vi "gu_free.vi"(8 "error in":errorcluster, 11 "pointer":i64) -> (0 "error out":errorcluster)   [LabVIEW 2020, in "G-Unicode.lvlib"]
doc: "Free the memory pointed to by <b>pointer</b>."
uses:
  G-Unicode.lvlib
  lib/g_unicode_32.dll
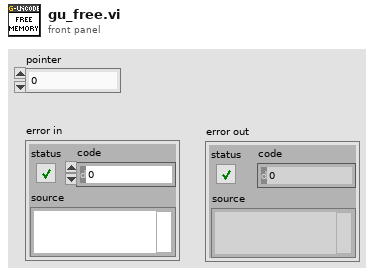
[diagram p1: front panel]
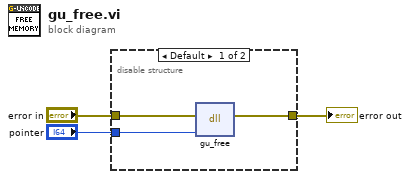
[diagram p0: block diagram]
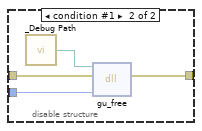
[diagram p2: hidden frame]
diagram:
  n1 = disable-structure shown="Default" {
    disable-tunnel: "pointer" -> [w6 w10]
    disable-tunnel: "error in" -> [w5 w9]
    disable-tunnel: [w4 w8] -> w1
    frame condition #0 (active) {
      n2 = dll-call lib="C:/github/dataflowg/g-unicode/src/LabVIEW/G-Unicode/lib/g_unicode_*.*" fn="gu_free"(error in=w5, "pointer"=w6) -> (error out=w4:errorcluster)  [unwired: 4 in, 1 out]
    }
    frame condition #1 {
      n3 = call "_Debug Path.vi"() -> ("Debug Path"=w7:path)
      n4 = dll-call lib="?" fn="gu_free"(path in=w7, error in=w9, "pointer"=w10) -> (error out=w8:errorcluster)  [unwired: 3 in, 1 out]
    }
  }
  "error out" <- w1
